vi "运行间隔计算.vi"(11 "运行周期":i16=4) -> (3 "数组":i32[](array[numeric]))   [LabVIEW 2016, in "流量计集成.lvlib" / "流量计.lvlib"]
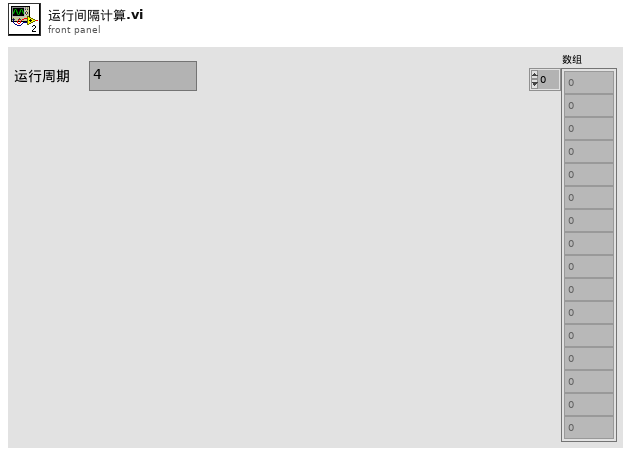
[diagram p1: front panel]
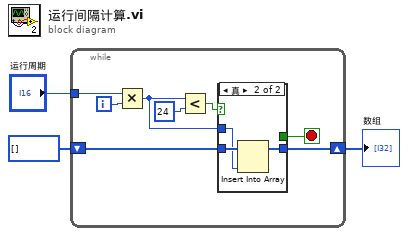
[diagram p0: block diagram]
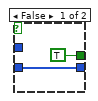
[diagram p2: hidden frame]
diagram:
  n1 = while {
    tunnel: "运行周期" -> [w11]
    shift-right: [w8] -> w1
    shift-left: i32[] [] -> [w9]
    i -> [w10]
    stop <- w5 stop-if-true
    n2 = Multiply(x=w11, y=w10) -> (x*y=w4:i32)
    n3 = Less?(x=w4, y=24) -> (x < y?=w6:bool)
    n4 = case shown="真" w6 {
      tunnel: w9 -> [w13 w16]
      tunnel: [w13 w15] -> w8
      tunnel: [TRUE _] -> w5
      tunnel: w4 -> [_ w14]
      frame False {
      }
      frame True {
        n5 = Insert Into Array(array=w16, new element=w14) -> (w15:i32[])  [unwired: 1 in]
      }
    }
  }
  "数组" <- w1
